vi "test_convert_settings.vi"() -> ()   [LabVIEW 2025]
uses:
  FPGA/fpga_settings.ctl
  <vilib>/rvi/FXPMathLib/FxpInterpret/XNode/nifxpmath_Interpret.xnode
  FPGA/subVIs/Setpoint type.ctl
panel:
  out "unsigned 16bit integer":u16
  in  "FPGA Setting":T1
  in  "Setpoint type":T2
  out "fixed-point":fxp<+/-,32,14>
  out "hi(x)":u16
  in  "Fixed I":fxp<+/-,32,14>
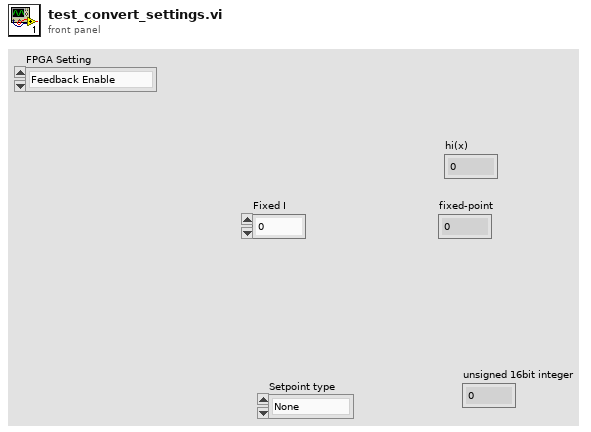
[diagram p1: front panel]
types:
  T1 = typedef "fpga_settings.ctl" = enum16{"Feedback Enable", "New FIR coeffs", "FIR shift", "Enable filter", "Set Downsample", "Downsample", "CIC Gain", "Record length", "Trigger samples", "Quiet time", "a_am", "b_am", "Use fixed delay", "fixed sin_fi", "fixed cos_fi", "Ki*Tau", "Kp", "Kd_Tau", "Fi_start", "Fi_delta", "DC_offs 0", "DC_offs 1", "DC_offs 2", "DC_offs 3", "Ki*Tau am", "Kp am", "Kd_Tau am", "Feedback AM", "Trigger delay", "Feedback delay", "Setpoint enable", "Beam enable", "Samples to acquire", "Cavity Enable", "Cavity C1", "Cavity C2", "Cavity C3", "Cavity C4", "Cavity C5", "Input delay", "Ki*Tau Q", "Kp Q", "Kd_Tau Q", "Adaptive FF enable", "Feedforward a0", "Feedforward b0", "FF src adress", "FF dest adress", "Output scale", "Input scale", "Host scale", "FF_IIR b0", "FF_IIR b1", "FF_IIR b2", "FF_IIR-a1", "FF_IIR-a2", "Enable HW trigger", "Virtual cavity", "Samples to skip", "Samples to skip 2", "Samples to skip 3", "Cavity C3_2", "Cavity C4_2", "Cavity C5_2", "Cavity C3_3", "Cavity C4_3", "Cavity C5_3", "Cavity_w0_dt", "Piezo setting", "Quench t0", "Quench tau set", "Quench enabled", "Quench reset", "PID enabled I", "PID enabled Q", "Cavity filter a", "Cavity filter b", "Disable e(n)", "FF e(n) src address", "FF first address", "FF last address", "FF PID first address", "FF PID last address", "Amp IIR b0", "Amp IIR b1", "Amp IIR b2", "Amp IIR-a1", "Amp IIR-a2", "Adaptation factor", "Inv Amp LP b0", "Inv Amp LP b1", "Inv Amp LP b2", "Inv Amp LP-a1", "Inv Amp LP-a2", "Inv Amp c0", "Inv Amp c1", "Inv Amp c2", "Inv Amp c3", "Inv Amp c4", "Inv Amp -d1", "Inv Amp -d2", "Inv Amp -d3", "Inv Amp -d4", "w12_a", "w12_b", "w12_dt", "w12_scale", "dw_scale", "Extra output select", "Extra fi sin", "Extra fi cos", "Extra output scale", "Quench max output", "Fixed SP I", "Fixed SP Q"}
  T2 = typedef "Setpoint type.ctl" = enum16{"None", "Memory", "Fixed"}
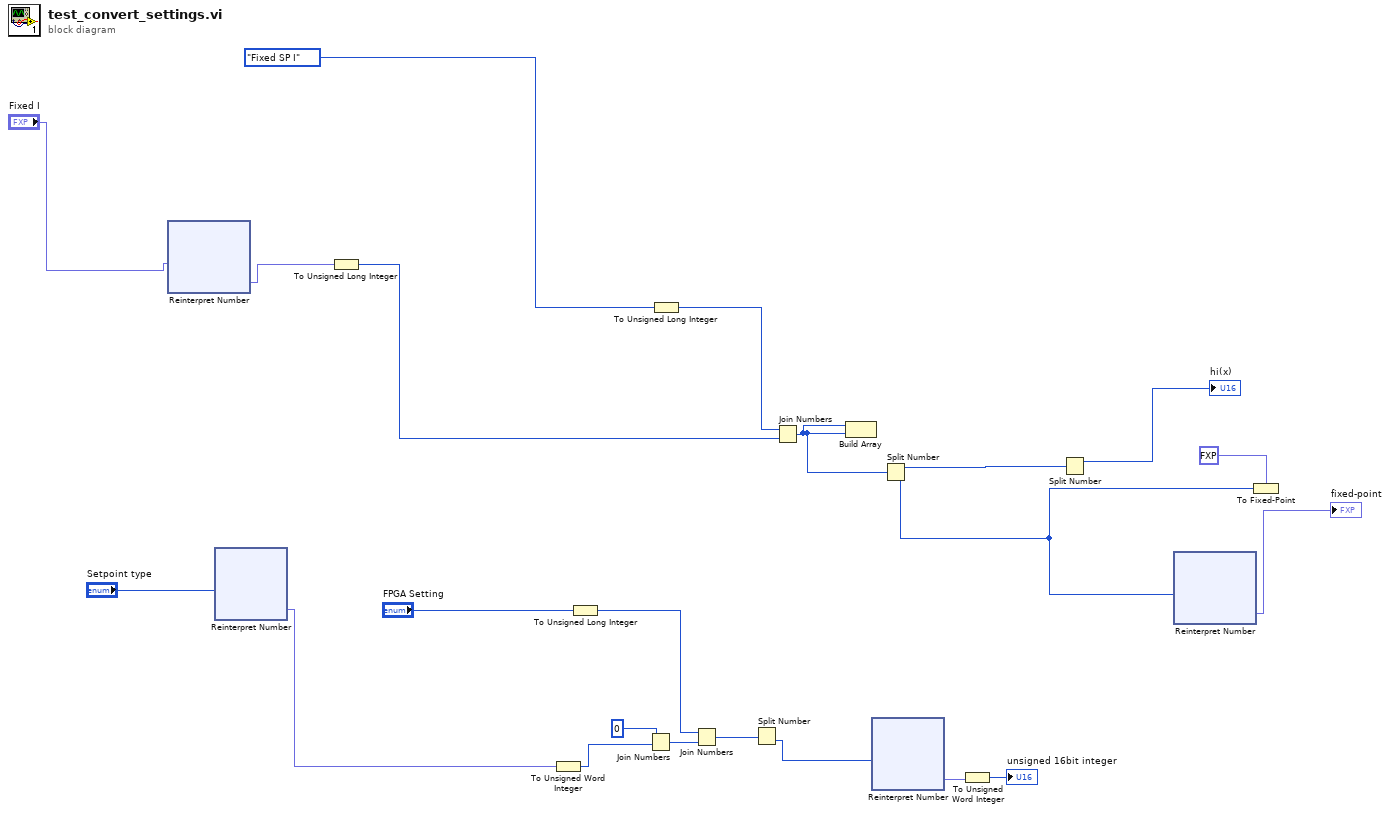
[diagram p0: block diagram]
diagram:
  n1 = xnode "Reinterpret Number"("x"="Fixed I") -> ("y"=w12:fxp<+,32,32>)
  n2 = xnode "Reinterpret Number"("x"="Setpoint type") -> ("y"=w5:fxp<+,16,16>)
  n3 = To Unsigned Long Integer(number=w12) -> (unsigned 32bit integer=w21:u32)
  n4 = To Unsigned Word Integer(number=w5) -> (unsigned 16bit integer=w8:u16)
  n5 = To Unsigned Long Integer(number="FPGA Setting") -> (unsigned 32bit integer=w6:u32)
  n6 = Join Numbers(hi=u16 0, lo=w8) -> ((hi.lo)=w9:u32)
  n7 = To Unsigned Long Integer(number=fpga_settings."Fixed SP I" ("FPGA Setting")) -> (unsigned 32bit integer=w22:u32)
  n8 = Join Numbers(hi=w6, lo=w9) -> ((hi.lo)=w3:u64)
  n9 = Split Number(x=w3) -> (lo(x)=w2:u32)  [unwired: 1 out]
  n10 = Join Numbers(hi=w22, lo=w21) -> ((hi.lo)=w17:u64)
  n11 = Build Array(w17, w17) -> ()  [unwired: 1 out]
  n12 = xnode "Reinterpret Number"("x"=w2) -> ("y"=w4:fxp<+,32,32>)
  n13 = Split Number(x=w17) -> (hi(x)=w19:u32, lo(x)=w15:u32)
  n14 = To Unsigned Word Integer(number=w4) -> (unsigned 16bit integer=→"unsigned 16bit integer":u16)
  n15 = Split Number(x=w19) -> (hi(x)=→"hi(x)":u16)  [unwired: 1 out]
  n16 = xnode "Reinterpret Number"("x"=w15) -> ("y"=→"fixed-point":fxp<+/-,32,14>)
  n17 = To Fixed-Point(fixed-point type=fxp<+/-,32,14> 0.0 ("Data"), number=w15) -> ()  [unwired: 1 out]
